vi "Initialize HMI.vi"(8 "error in (no error)":errorcluster, 11 "Device Name":string="Logitech Extreme 3D" caption="Give the exact \"divice name\" string of the joypad you would like to use.") -> (0 "error out":errorcluster, 3 "Device":T1={"device ID"=refnum, "Device Name"="Logitech Extreme 3D", "axis info"={"X axis"=[], "Y axis"=[], "Z axis"=[], "X axis rotation"=[], "Y axis rotation"=[], "Z axis rotation"=[], "U axis"=[], "V axis"=[]}}, 5 "Listed Devices":T2(array[cluster]))   [LabVIEW 2012]
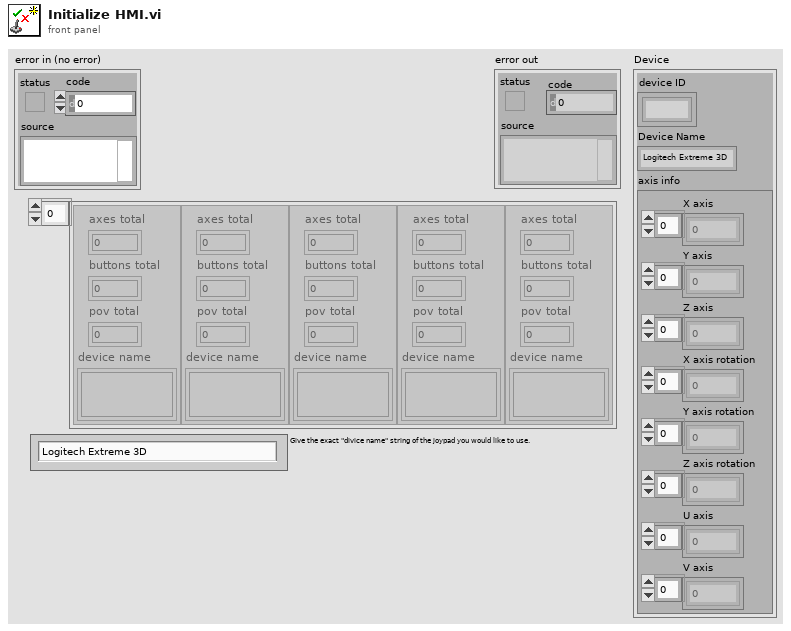
[diagram p1: front panel]
types:
  T1 = cluster{"device ID":refnum<k1>, "Device Name":string, "axis info":cluster{"X axis":dbl[], "Y axis":dbl[], "Z axis":dbl[], "X axis rotation":dbl[], "Y axis rotation":dbl[], "Z axis rotation":dbl[], "U axis":dbl[], "V axis":dbl[]}}
  T2 = cluster{"axes total":u32, "buttons total":u32, "pov total":u32, "device name":string}[]
  T3 = cluster{"X axis":dbl[], "Y axis":dbl[], "Z axis":dbl[], "X axis rotation":dbl[], "Y axis rotation":dbl[], "Z axis rotation":dbl[], "U axis":dbl[], "V axis":dbl[]}
  T4 = cluster{"X axis":i32, "Y axis":i32, "Z axis":i32, "X axis rotation":i32, "Y axis rotation":i32, "Z axis rotation":i32, "U axis":i32, "V axis":i32}
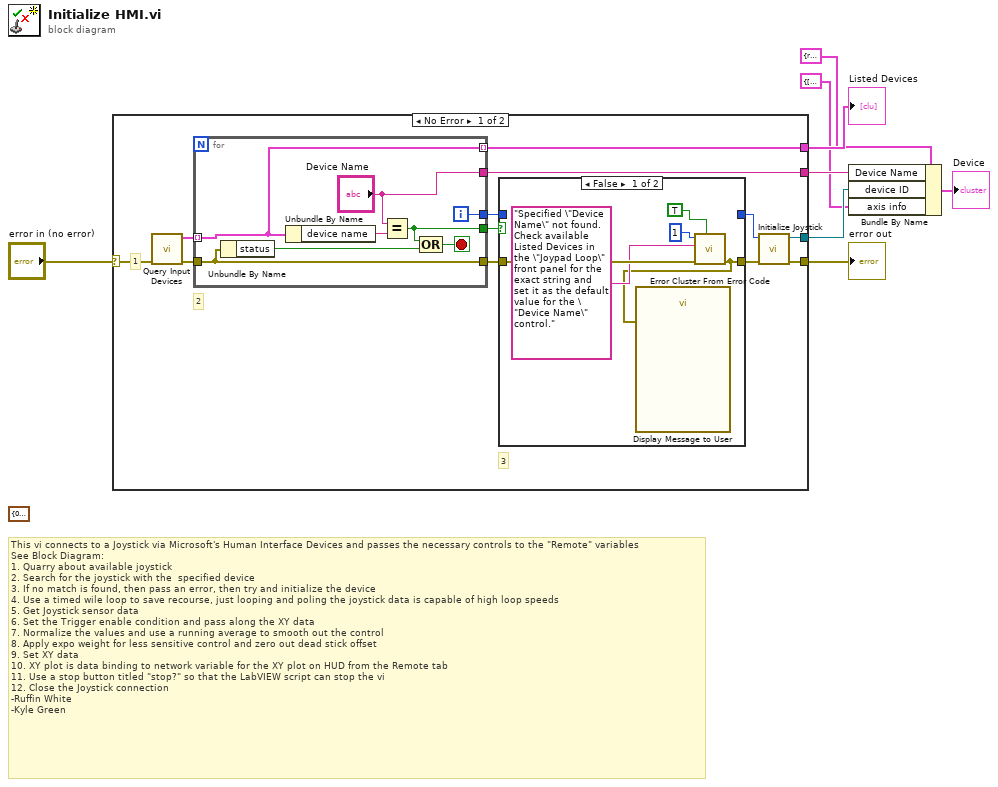
[diagram p0: block diagram]
diagram:
  (unwired) T4 {"X axis"=0, "Y axis"=0, "Z axis"=0, "X axis rotation"=0, "Y axis rotation"=0, "Z axis rotation"=0, "U axis"=0, "V axis"=0} ("axis info")
  # "This vi connects to a Joystick via Microsoft's Human Interface Devices and passes the necessary controls to the \"Remote\" variables   \nSee Block Diagram:\n1.\tQuarry about available joystick\n2.\tSearch for the joystick with the  specified device\n3.\tIf no match is found, then pass an error, then try and initialize the device\n4.\tUse a timed wile loop to save recourse, just looping and poling the joystick data is capable of high loop speeds\n5.\tGet Joystick sensor data\n6.\tSet the Trigger enable condition and pass along the XY data\n7.\tNormalize the values and use a running average to smooth out the control\n8.\tApply expo weight for less sensitive control and zero out dead stick offset \n9.\tSet XY data\n10.\tXY plot is data binding to network variable for the XY plot on HUD from the Remote tab\n11.\tUse a stop button titled \"stop?\" so that the LabVIEW script can stop the vi\n12.\tClose the Joystick connection\n-Ruffin White\n-Kyle Green"
  n1 = case shown="No Error" "error in (no error)" {
    selector: "error in (no error)" -> [w9 w36]
    tunnel: [w15 _] -> w8
    tunnel: [w12 w36] -> w7
    tunnel: [w11 _] -> w5
    tunnel: [w10 _] -> w4
    frame No Error {
      # "3"
      # "2"
      # "1"
      n2 = call <vilib>:"Query Input Devices.vi"("error in (no error)"=w9) -> ("error out"=w17:errorcluster, "joystick info"=w20:T2)  [unwired: 7 in, 2 out]
      n3 = for {
        tunnel: w20 -> [w29] mode=indexing
        tunnel: [w34] -> w19
        tunnel: [w31] -> w18
        tunnel: w17 -> [w32]
        tunnel: [w32] -> w16
        tunnel: [w29] -> w15 mode=indexing
        tunnel: ["Device Name"] -> w10
        i -> [w34]
        stop <- w33 stop-if-true
        n4 = Unbundle By Name(w32) -> ("status"=w30:bool)
        n5 = Unbundle By Name(w29) -> ("device name"=w35:string)
        n6 = Equal?(x="Device Name", y=w35) -> (x = y?=w31:bool)
        n7 = Compound Arithmetic op=OR(w31, w30) -> (w33:bool)
      }
      n8 = case shown="False" w18 {
        tunnel: w19 -> [_ w27]
        tunnel: [_ w27] -> w14
        tunnel: w16 -> [w25 w26]
        tunnel: [w21 w26] -> w13
        frame False {
          n9 = call <vilib>:"Error Cluster From Error Code.vi"("show call chain? (False)"=TRUE, "error in (no error)"=w25, "error message (\"\")"="Specified \"Device Name\" not found. Check available Listed Devices in the \"Joypad Loop\" front panel for the exact string and set it as the default value for the \"Device Name\" control." ("error message (\"\")"), "error code (0)"=1) -> ("error out"=w21:errorcluster)  [unwired: 5 in]
          n10 = call "Display Message to User"("error in (no error)"=w21) -> ()  [unwired: 9 in, 2 out]
        }
        frame True {
        }
      }
      n11 = call <vilib>:"Initialize Joystick.vi"("error in (no error)"=w13, "device index"=w14) -> ("error out"=w12:errorcluster, "device ID"=w11:refnum<k1>)  [unwired: 8 in]
    }
    frame Error {
    }
  }
  "Listed Devices" <- w8
  "error out" <- w7
  n12 = Bundle By Name(cluster=T1 {"device ID"=refnum, "Device Name"="Logitech Extreme 3D", "axis info"={"X axis"=[], "Y axis"=[], "Z axis"=[], "X axis rotation"=[], "Y axis rotation"=[], "Z axis rotation"=[], "U axis"=[], "V axis"=[]}} ("Device"), "Device Name"=w4, "device ID"=w5, "axis info"=T3 {"X axis"=[0.0, 0.0], "Y axis"=[0.0, 0.0], "Z axis"=[0.0, 0.0], "X axis rotation"=[0.0, 0.0], "Y axis rotation"=[0.0, 0.0], "Z axis rotation"=[0.0, 0.0], "U axis"=[0.0, 0.0], "V axis"=[0.0, 0.0]}) -> (→"Device":T1)
